vi "all_settings_to_string.vi"(5 "Analog Output Parameters":T9={"Enable Analog Out?"=TRUE, "Physical Channel"="PXI1Slot2/ao0:3", "Minimum Value"=-10.0, "Maximum Value"=10.0, "Samples per second"=10000.0, "Total AO Time (seconds)"=0.0, "Start Trigger"={"Wait for start trigger?"=FALSE, "source"="/Dev1/PFI0", "edge"=10280}, "Analog Output Waveforms (channel, time)"=[], "Export trigger"={"Export Start Trigger?"=FALSE, "output terminal"=""}} {"Start Trigger"."edge" items=["Rising"=10280, "Falling"=10171]; "Maximum Value" format="%0.2f"; "Minimum Value" format="%0.2f"}, 7 "Camera Setup":T8={"Analog Gain (0-5)"=4, "Exposure Time"=0.01, "EM Gain (0-255)"=0, "Trigger Polarity"="ATP P", "External Trigger Mode"="ATP P", "Scan Speed"="EMD E", "External Trigger Source"="SSP H", "Scan Mode"="ESC B", "Super Pixel Binning\n(if enabled in Scan Mode)"="SMD N", "Camera Sub-array acquisition region\n(if enabled in scan mode)"={"Left"=0, "Top"=0, "Width"=0, "Height"=0}, "Use camera?"=FALSE, "# image buffers"=100, "shots per measurement"=100, "Force images to U16"=FALSE, "Low Light Sensitivity"="LLS 0", "cooling"="CSW F", "fan"="FAN F", "Frame Grabber acquisition region"={"Left"=0, "Top"=0, "Right"=0, "Bottom"=0}} {"Frame Grabber acquisition region"."Bottom" max=512 step=1; "Frame Grabber acquisition region"."Right" max=512 step=1; "Frame Grabber acquisition region"."Top" max=512 step=1; "Frame Grabber acquisition region"."Left" max=512 step=1; "shots per measurement" min=0 step=1; "# image buffers" min=0 step=1; "Camera Sub-array acquisition region\n(if enabled in scan mode)"."Height" min=16 max=512 step=16; "Camera Sub-array acquisition region\n(if enabled in scan mode)"."Width" min=16 max=512 step=16; "Camera Sub-array acquisition region\n(if enabled in scan mode)"."Top" max=496 step=16; "Camera Sub-array acquisition region\n(if enabled in scan mode)"."Left" max=496 step=16; "Analog Gain (0-5)" max=5 step=1}, 8 "error in":errorcluster, 10 "HSDIO Settings":T1={"Enable HSDIO Pulses"=TRUE, "Resource Name"="PXI1Slot6", "Clock Rate"=20000000.0, "Array of Script Triggers"=[], "Pulse Generation Script"="script script1\n     wait 1\nend script", "Start Trigger"={"Wait for start trigger?"=FALSE, "source (PFI 0)"="PFI0", "edge (rising)"=12, "description"=""}, "Hardware alignment quantum\n(in samples)"=1, "Inital State"="", "Idle State"="", "Active Channels"="", "Array of Waveforms"=[], "description"=""} {"Hardware alignment quantum\n(in samples)" min=1 step=1; "Array of Script Triggers"."level" items=["High Level"=34, "Low Level"=35]; "Array of Script Triggers"."edge" items=["Rising Edge"=12, "Falling Edge"=13]; "Start Trigger"."edge (rising)" items=["Rising Edge"=12, "Falling Edge"=13]; "Clock Rate" min=0.0 max=200000000.0 format="%.2p"}, 11 "Variable Settings":T7={"Measurements per Iteration"=1, "Local Data Path"=path "C:/Users/Saffmanlab/Documents/Cesium/data", "Experiment description suffix for filename (no spaces please)"="", "Network Data Path"=path "Z:/", "Copy data to network"=TRUE, "Measurement Timeout (ms)"=0, "Variables"=[], "Parameters"=[], "Run Test Mode"=FALSE} {"Variables"."# steps" min=1 step=1; "Measurements per Iteration" min=1 step=1}) -> (0 "error out":errorcluster, 1 "all settings string":string)   [LabVIEW 2013]
uses:
  Analog_output/Analog_Output.lvclass
  ExperimentVariables/ExperimentVariables.lvclass
  HSDIO/HSDIO.lvclass
  Analog_output/AO_settings.ctl
  Camera/Hamamatsu_C9100-13/camera_setup.ctl
  Camera/Hamamatsu_C9100-13/Hamamatsu_C9100-13.lvclass
  ExperimentVariables/Variable_Settings.ctl
  <instrlib>/niHSDIO/niHSDIO.llb/niHSDIO_ctl Trigger Source Values (Ring).ctl
  <instrlib>/niHSDIO/niHSDIO.llb/niHSDIO_ctl Trigger DigEdge - Edge Values (Ring).ctl
  <instrlib>/niHSDIO/niHSDIO.llb/niHSDIO_ctl Trigger Script - trigID Values (Ring).ctl
  <instrlib>/niHSDIO/niHSDIO.llb/niHSDIO_ctl Trigger DigLvl - Level Values (Ring).ctl
  HSDIO/HSDIO_settings.ctl
  HSDIO/waveform.ctl
panel:
  # "Parameters will be evaluated once at the beginning of the experiment from top to bottom, \nso any parameter may depend on all those above it.\nVariables will be evaluated each iteration.\nParameters and Variables may be used in various other experiment settings, as noted.\nSee LabView Help -> Formula Node and Expression Node Functions for a list of available functions."
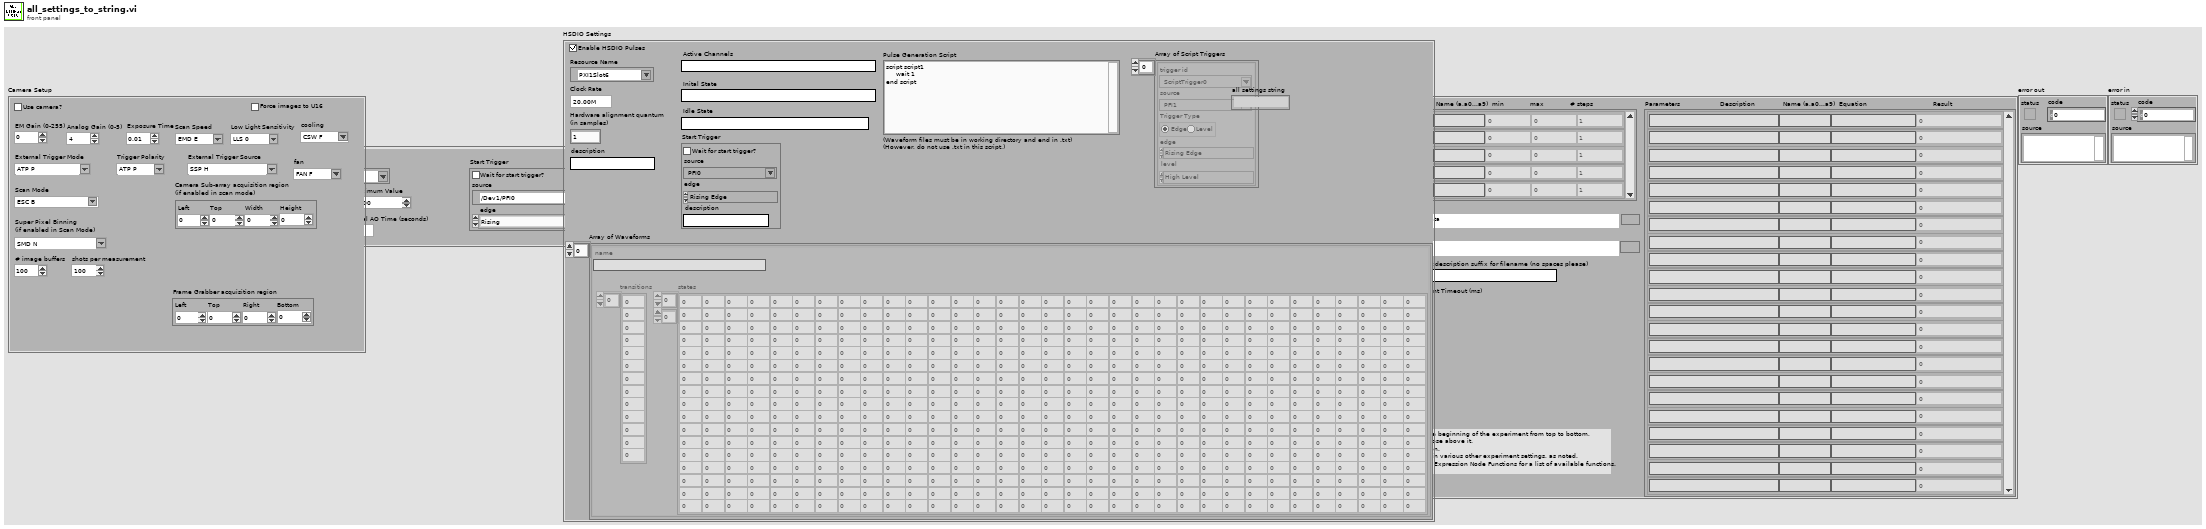
[diagram p1: front panel]
types:
  T1 = typedef "HSDIO.lvclass/HSDIO_settings.ctl" = cluster{"Enable HSDIO Pulses":bool, "Resource Name":refnum<k15>, "Clock Rate":dbl, "Array of Script Triggers":cluster{"trigger id (script trigger 0)":T2, "source (PFI 0)":T3, "Trigger Type":enum32{"Edge", "Level"}, "edge":T4, "level":T5}[], "Pulse Generation Script":string, "Start Trigger":cluster{"Wait for start trigger?":bool, "source (PFI 0)":T3, "edge (rising)":T4, "description":string}, "Hardware alignment quantum\n(in samples)":u16, "Inital State":string, "Idle State":string, "Active Channels":string, "Array of Waveforms":T6[], "description":string}
  T2 = typedef "niHSDIO_ctl Trigger Script - trigID Values (Ring).ctl" = string
  T3 = typedef "niHSDIO_ctl Trigger Source Values (Ring).ctl" = string
  T4 = typedef "niHSDIO_ctl Trigger DigEdge - Edge Values (Ring).ctl" = i32
  T5 = typedef "niHSDIO_ctl Trigger DigLvl - Level Values (Ring).ctl" = i32
  T6 = typedef "HSDIO.lvclass/waveform.ctl" = cluster{"name":string, "transitions":u32[], "states":u8[][]}
  T7 = typedef "ExperimentVariables.lvclass/Variable_Settings.ctl" = cluster{"Measurements per Iteration":i32, "Local Data Path":path, "Experiment description suffix for filename (no spaces please)":string, "Network Data Path":path, "Copy data to network":bool, "Measurement Timeout (ms)":u32, "Variables":cluster{"Description":string, "Name (a,a0...a9)":string, "min":dbl, "max":dbl, "# steps":u32}[], "Parameters":cluster{"Description":string, "Name (a,a0...a9)":string, "Equation":string, "Result":dbl}[], "Run Test Mode":bool}
  T8 = typedef "Hamamatsu_C9100-13.lvclass/camera_setup.ctl" = cluster{"Analog Gain (0-5)":u8, "Exposure Time":dbl, "EM Gain (0-255)":u8, "Trigger Polarity":string, "External Trigger Mode":string, "Scan Speed":string, "External Trigger Source":string, "Scan Mode":string, "Super Pixel Binning\n(if enabled in Scan Mode)":string, "Camera Sub-array acquisition region\n(if enabled in scan mode)":cluster{"Left":u16, "Top":u16, "Width":u16, "Height":u16}, "Use camera?":bool, "# image buffers":i32, "shots per measurement":i32, "Force images to U16":bool, "Low Light Sensitivity":string, "cooling":string, "fan":string, "Frame Grabber acquisition region":cluster{"Left":i32, "Top":i32, "Right":i32, "Bottom":i32}}
  T9 = typedef "Analog_Output.lvclass/AO_settings.ctl" = cluster{"Enable Analog Out?":bool, "Physical Channel":tag, "Minimum Value":dbl, "Maximum Value":dbl, "Samples per second":dbl, "Total AO Time (seconds)":dbl, "Start Trigger":cluster{"Wait for start trigger?":bool, "source":tag, "edge":i32}, "Analog Output Waveforms (channel, time)":dbl[][], "Export trigger":cluster{"Export Start Trigger?":bool, "output terminal":tag}}
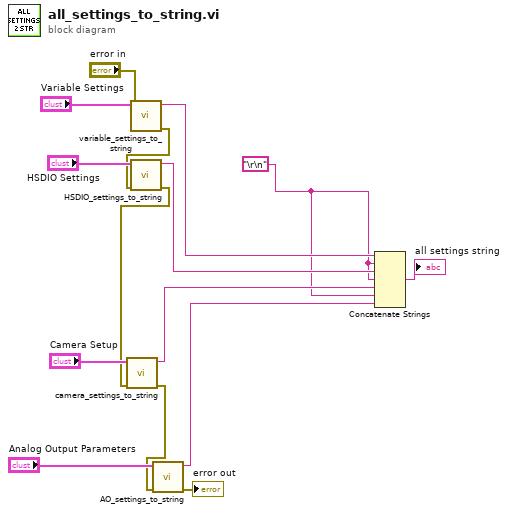
[diagram p0: block diagram]
diagram:
  w2 = "\r\n"
  n1 = call "variable_settings_to_string.vi"("error in"="error in", "Variable Settings"="Variable Settings") -> ("error out"=w11:errorcluster, "varible settings string"=w5:string)  [unwired: 8 in]
  n2 = call "HSDIO_settings_to_string.vi"("error in"=w11, "HSDIO Settings"="HSDIO Settings") -> ("error out"=w9:errorcluster, "resulting string"=w4:string)  [unwired: 8 in]
  n3 = call "camera_settings_to_string.vi"("error in"=w9, "Camera Setup"="Camera Setup") -> ("error out"=w8:errorcluster, "Camera Setup string"=w3:string)  [unwired: 8 in]
  n4 = call "AO_settings_to_string.vi"("error in"=w8, "Analog Output Parameters"="Analog Output Parameters") -> ("error out"=→"error out":errorcluster, "Analog Output Settings string"=w1:string)  [unwired: 8 in]
  n5 = Concatenate Strings(w5, w2, w4, w2, w3, w2, w1) -> (→"all settings string":string)
